vi "Main.vi"() -> ()   [LabVIEW 2018, in "Filter Pattern Demo.lvclass"]
uses:
  Filter Pattern Demo.lvclass
  Person Class/Person.lvclass
  AndCriteria Class/AndCriteria.lvclass
  C:/Users/fflores/Documents/LabVIEW-Open-Projects/LabIVEW OOP Design Patterns/Filter Pattern/Criteria Class/Criteria.lvclass
  OrCriteria Class/OrCriteria.lvclass
  CriteriaMale Class/CriteriaMale.lvclass
  CriteriaSingle Class/CiteriaSingle.lvclass
  CriteriaFemale Class/CriteriaFemale.lvclass
  ConsoleOut/Print Options.ctl
  Criteria Class/Criteria.lvclass
panel:
  out "error out":errorcluster
  in  "Raw Data":string[][](table)=[["Robert", "Male", "Single"], ["John", "Male", "Married"], ["Laura", "Female", "Married"], ["Diana", "Female", "Single"], ["Mike", "Male", "Single"], ["Bobby", "Male", "Single"]]
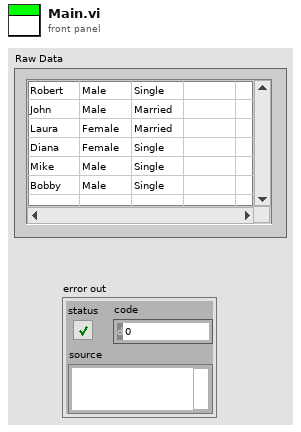
[diagram p1: front panel]
types:
  T1 = typedef "Print Options.ctl" = enum16{"Create", "Get Reference", "Print", "Print Header", "Close"}
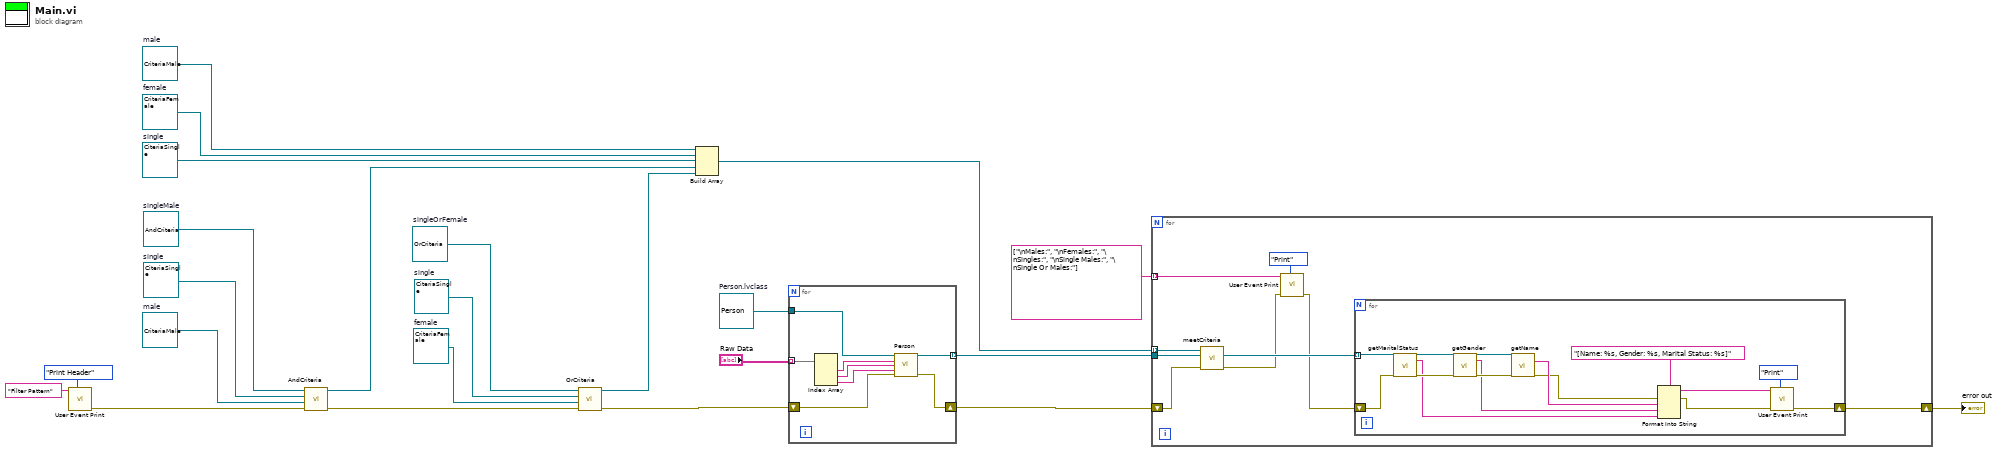
[diagram p0: block diagram]
diagram:
  w17 = refnum<class "CriteriaFemale.lvclass"> refnum  # female
  w18 = refnum<class "CiteriaSingle.lvclass"> refnum  # single
  w19 = refnum<class "CriteriaMale.lvclass"> refnum  # male
  w20 = refnum<class "CiteriaSingle.lvclass"> refnum  # single
  w22 = refnum<class "OrCriteria.lvclass"> refnum  # singleOrFemale
  w21 = refnum<class "AndCriteria.lvclass"> refnum  # singleMale
  w13 = refnum<class "CiteriaSingle.lvclass"> refnum  # single
  w14 = refnum<class "CriteriaFemale.lvclass"> refnum  # female
  w15 = refnum<class "CriteriaMale.lvclass"> refnum  # male
  w23 = refnum<class "Person.lvclass"> refnum  # Person.lvclass
  n1 = call "User Event Print.vi"("Options"=Print_Options."Print Header", "String to Print"="Filter Pattern") -> ("error out"=w4:errorcluster)  [unwired: 8 in, 1 out]
  n2 = call "AndCriteria.vi"("error in (no error)"=w4, "Other Criteria"=w19, "Criteria"=w20, "AndCriteria in"=w21) -> ("error out"=w3:errorcluster, "AndCriteria out"=w12:refnum<class "AndCriteria.lvclass">)  [unwired: 6 in]
  n3 = call "OrCriteria.vi"("error in (no error)"=w3, "Other Criteria"=w17, "Criteria"=w18, "OrCriteria in"=w22) -> ("error out"=w2:errorcluster, "OrCriteria out"=w11:refnum<class "OrCriteria.lvclass">)  [unwired: 6 in]
  n4 = Build Array(w15, w14, w13, w12, w11) -> (w10:refnum<class "Criteria.lvclass">[])
  n5 = for {
    tunnel: "Raw Data" -> [w31] mode=indexing
    tunnel: w23 -> [w27]
    tunnel: [w26] -> w9 mode=indexing
    shift-right: [w24] -> w5
    shift-left: w2 -> [w25]
    n6 = Index Array(array=w31) -> (element #1=w30:string, element #2=w29:string, element #3=w28:string)  [unwired: 3 in]
    n7 = call "Person.vi"("Person in"=w27, "name"=w30, "gender"=w29, "maritalStatus"=w28, "error in (no error)"=w25) -> ("Person out"=w26:refnum<class "Person.lvclass">, "error out"=w24:errorcluster)  [unwired: 9 in]
  }
  n8 = for {
    tunnel: w10 -> [w40] mode=indexing
    tunnel: w9 -> [w39]
    tunnel: string[] ["\nMales:", "\nFemales:", "\nSingles:", "\nSingle Males:", "\nSingle Or Males:"] -> [w35] mode=indexing
    shift-right: [w32] -> w1
    shift-left: w5 -> [w33]
    n9 = call-dynamic "meetCriteria.vi"("error in (no error)"=w33, "Persons In"=w39, "Criteria in"=w40) -> ("error out"=w37:errorcluster, "Persons Out"=w38:refnum<class "Person.lvclass">[])  [unwired: 6 in, 1 out]
    n10 = call "User Event Print.vi"("Options"=Print_Options."Print", "error in (no error)"=w37, "String to Print"=w35) -> ("error out"=w36:errorcluster)  [unwired: 7 in, 1 out]
    n11 = for {
      tunnel: w38 -> [w51] mode=indexing
      shift-right: [w41] -> w32
      shift-left: w36 -> [w46]
      n12 = call-dynamic "getMaritalStatus.vi"("error in (no error)"=w46, "Person in"=w51) -> ("error out"=w54:errorcluster, "maritalStatus"=w47:string, "Person out"=w55:refnum<class "Person.lvclass">)  [unwired: 7 in]
      n13 = call-dynamic "getGender.vi"("error in (no error)"=w54, "Person in"=w55) -> ("error out"=w52:errorcluster, "gender"=w48:string, "Person out"=w53:refnum<class "Person.lvclass">)  [unwired: 7 in]
      n14 = call-dynamic "getName.vi"("error in (no error)"=w52, "Person in"=w53) -> ("error out"=w43:errorcluster, "name"=w49:string)  [unwired: 7 in, 1 out]
      n15 = Format Into String(format string="[Name: %s, Gender: %s, Marital Status: %s]", error in=w43, w49, w48, w47) -> (resulting string=w44:string, error out=w42:errorcluster)  [unwired: 1 in]
      n16 = call "User Event Print.vi"("Options"=Print_Options."Print", "error in (no error)"=w42, "String to Print"=w44) -> ("error out"=w41:errorcluster)  [unwired: 7 in, 1 out]
    }
  }
  "error out" <- w1
